vi "ClassPanel.vi"(8 "error in (no error)":errorcluster caption="entrée d'erreur (pas d'erreur)", 11 "SR830.lvclass":refnum<class "SR830.lvclass">) -> (0 "error out":errorcluster caption="sortie d'erreur", 3 "SR830.lvclass Out":refnum<class "SR830.lvclass">)   [LabVIEW 2019, in "SR830.lvclass"]
uses:
  SR830.lvclass
  C:/Programmes Labview/LabScanV1A/DevicesClass/BaseDevice/BaseDevice.lvclass
  BaseDevice/BaseDevice.lvclass/BaseDevice.ctl
  BaseDevice/Accessor/GetBeforewait(ms).vi
  BaseDevice/Accessor/GetClassEvent.vi
  BaseDevice/Accessor/SetBeforewait.vi
panel:
  in  "MainProgQ":refnum<queue>
  in  "MainProgQEvent":refnum<user-event>
  in  "Time Constant":u16(ring)=1 items=["10 us", "30 us", "100 us", "300 us", "1 ms", "3 ms", "10 ms", "30 ms", "100 ms", "300 ms", "1 s", "3 s", "10 s", "30 s", "100 s", "300 s", "1 ks", "3 ks", "10 ks", "30 ks"]
  in  "BefWait (ms)":u32 caption="BeforeWait Delay(ms)" max=200000 step=1
  in  "Sensitivity":u16(ring)=1 items=["2 nV/fA", "5 nV/fA", "10 nV/fA", "20 nV/fA", "50 nV/fA", "100 nV/fA", "200 nV/fA", "500 nV/fA", "1 µV/pA", "2 µV/pA", "5 µV/pA", "10 µV/pA", "20 µV/pA", "50 µV/pA", "100µV/pA", "200 µV/pA", "500µV/pA", "1 mV/nA", "2 mV/nA", "5 mV/nA", "10 mV/nA", "20 mV/nA", "50 mV/nA", "100 mV/nA", "200 mV/nA", "500 mV/nA", "1 V/uA"]
  in  "Acq":bool
  out "Phase":dbl=1000.0 caption="Phase (°)" min=0.0 step=0.1 format="%#_5f"
  out "MAG":dbl=1000.0 caption="MAG (V)" min=0.0 step=0.1 format="%^#_6e"
  out "UNLCK":bool caption="SpexMov"
  out "X":dbl=1000.0 caption="X (V)" min=0.0 step=0.1 format="%^#_6e"
  in  "Stop":bool
  out "Init Program":bool
  out "OVLD":bool caption="SpexMov"
  in  "Update":bool caption="stopSpectro"
  out "Y":dbl=1000.0 caption="Y (V)" min=0.0 step=0.1 format="%^#_6e"
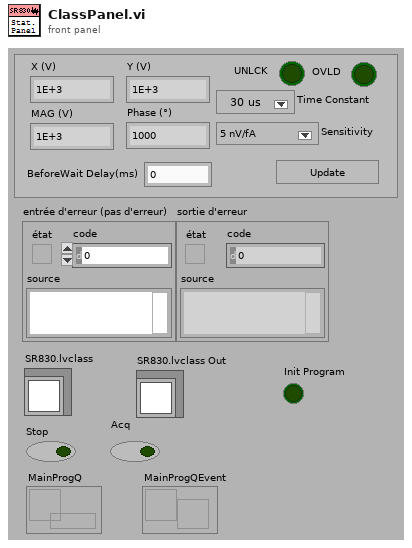
[diagram p1: front panel]
types:
  T1 = enum16{"Phase Shift", "Reference Source", "Reference Frequency", "Reference Trigger", "Detection Harmonic", "Sine Amplitude", "Input Configuration", "Input Shield", "Input Coupling", "Input Line Notch Filter", "Sensitivity", "Dynamic Reserve", "Time Constant", "Low Pass Filter", "Sync Filter", "Expand X", "Expand Y", "Expand R", "All"}
  T2 = enum16{"Sensitivity", "Dynamic Reserve", "Time Constant"}
  T3 = cluster{"Channels":u16, "Outputs":dbl[], "Status Byte":bool[]}
  T4 = enum8{"Enabled", "Disabled", "Disabled and Grayed Out"}
  T5 = cluster{"Phase Shift (°)":dbl, "Reference Source":u16, "Frequency (Hz)":dbl, "Reference Trigger":u16, "Harmonic":i32, "Sine Amplitude (V)":dbl, "Input Configuration":u16, "Input Shield":u16, "Input Coupling":u16, "Input Notch Filters":cluster{"1xLineFilter":bool, "2xLineFilter":bool}, "Sensitivity":u16, "Dynamic Reserve":u16, "Time Constant":u16, "Low Pass Filter":u16, "Sync Filter":bool, "Expand X":cluster{"Offset (%)":dbl, "Expand":u16}, "Expand Y":cluster{"Offset (%)":dbl, "Expand":u16}, "Expand R":cluster{"Offset (%)":dbl, "Expand":u16}}
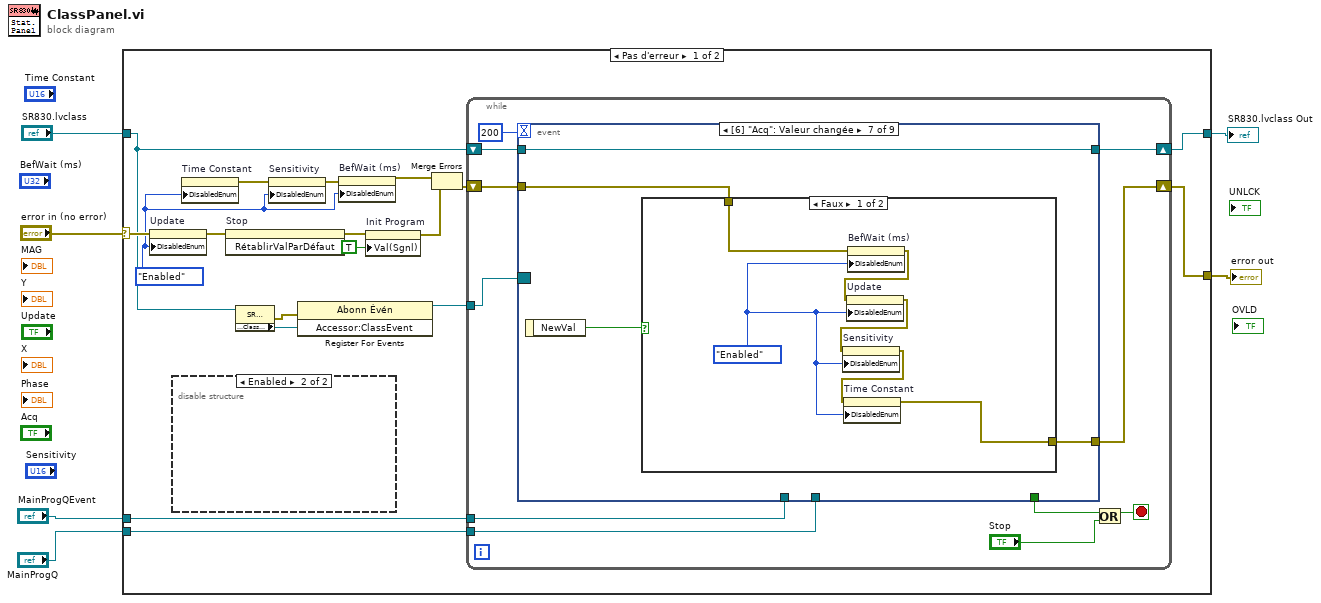
[diagram p0: block diagram]
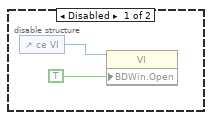
[diagram p2: hidden frame]
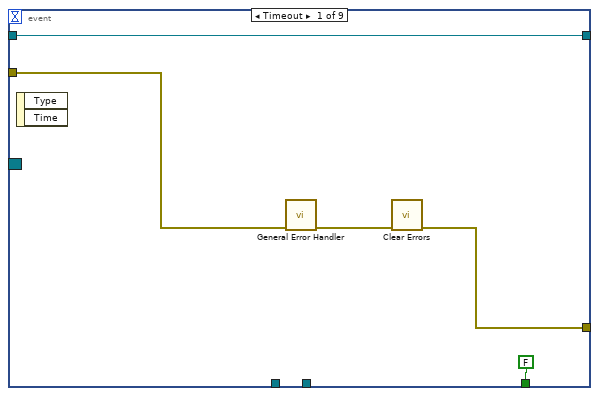
[diagram p3: hidden frame]
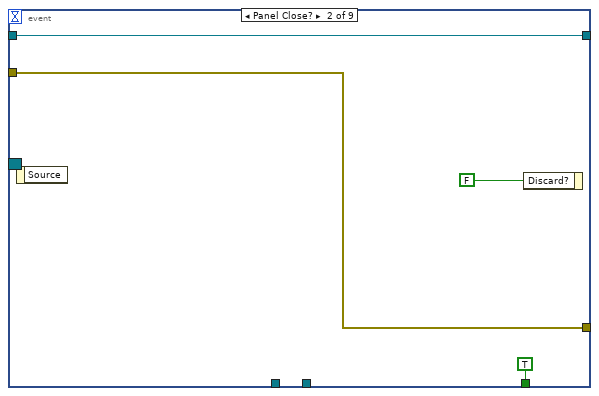
[diagram p4: hidden frame]
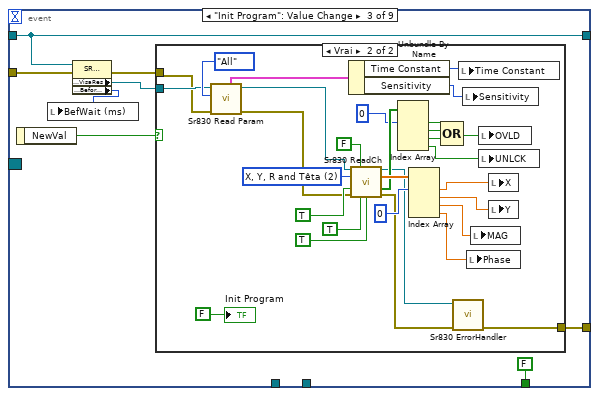
[diagram p5: hidden frame]
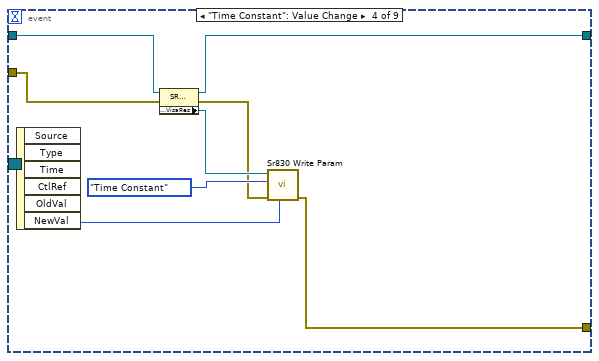
[diagram p7: hidden frame]
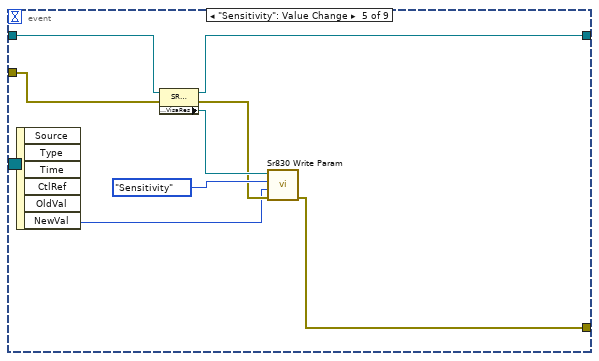
[diagram p8: hidden frame]
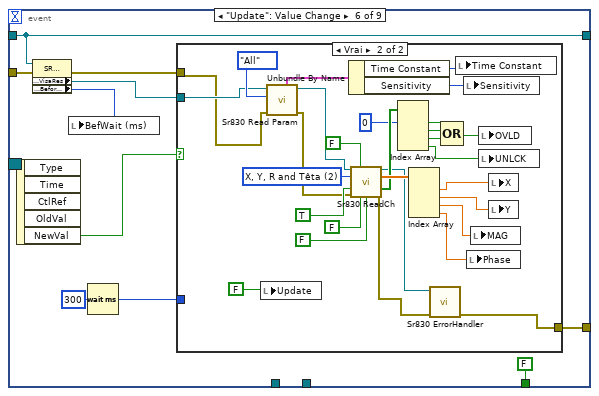
[diagram p9: hidden frame]
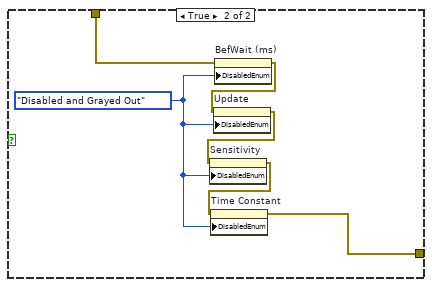
[diagram p11: hidden frame]
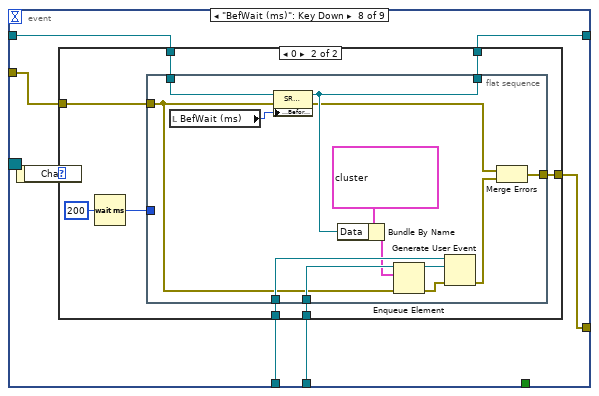
[diagram p12: hidden frame]
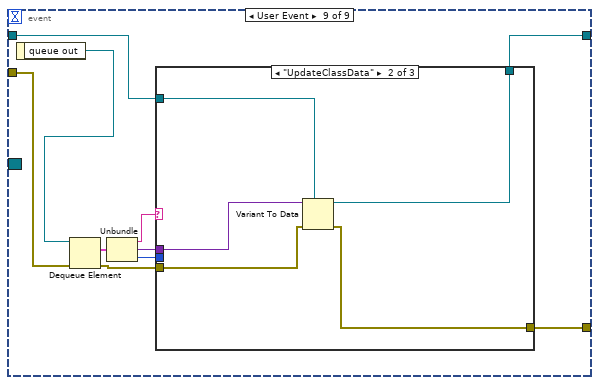
[diagram p14: hidden frame]
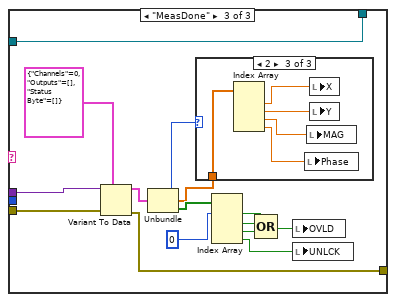
[diagram p16: hidden frame]
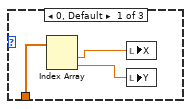
[diagram p17: hidden frame]
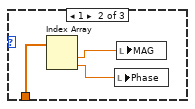
[diagram p18: hidden frame]
diagram:
  n1 = case shown="Pas d'erreur" "error in (no error)" {
    selector: "error in (no error)" -> [w21 w231]
    tunnel: [w16 w231] -> w5
    tunnel: "SR830.lvclass" -> [w14 w230]
    tunnel: [w23 w230] -> w3
    tunnel: "MainProgQEvent" -> [w13 _]
    tunnel: "MainProgQ" -> [w12 _]
    frame No Error {
      w7 = T4."Enabled" ("Désactivé")
      n2 = property on="Update" class="Bool (strict)"(error in=w21, "DisabledEnum"=w7) -> (error out=w18:errorcluster)  [unwired: 1 in, 1 out]
      n3 = disable-structure shown="Enabled" {
        frame Disabled {
          n4 = control-ref of="ce VI"() -> (w26:refnum<vi>)
          n5 = property class="VI"(reference=w26, "BDWin.Open"=TRUE ("Fenêtre du diagramme : ouverte")) -> ()  [unwired: 1 in, 2 out]
        }
        frame Enabled {
        }
      }
      n6 = property on="Time Constant" class="MDér (strict)"("DisabledEnum"=w7) -> (error out=w11:errorcluster)  [unwired: 2 in, 1 out]
      n7 = invoke on="Stop" class="Bool (strict)" method="RétablirValParDéfaut"(error in=w18) -> (error out=w22:errorcluster)  [unwired: 2 in, 2 out]
      n8 = property class="SR830.lvclass"(reference=w14) -> (error out=w19:errorcluster, "Accessor:ClassEvent"=w20:refnum<user-event>)  [unwired: 1 in, 1 out]
      n9 = property on="Sensitivity" class="MDér (strict)"(error in=w11, "DisabledEnum"=w7) -> (error out=w10:errorcluster)  [unwired: 1 in, 1 out]
      n10 = register-events(error in=w19, w20) -> (reference out=w17:refnum<event-registration>)  [unwired: 1 in, 1 out]
      n11 = property on="BefWait (ms)" class="NumNb (strict)"(error in=w10, "DisabledEnum"=w7) -> (error out=w8:errorcluster)  [unwired: 1 in, 1 out]
      n12 = property on="Init Program" class="Bool (strict)"(error in=w22, "Val(Sgnl)"=TRUE ("Valeur (Signalisation)")) -> (error out=w15:errorcluster)  [unwired: 1 in, 1 out]
      n13 = Merge Errors(w8, w15) -> (w9:errorcluster)
      n14 = while {
        shift-right: [w35] -> w16
        shift-left: w9 -> [w36]
        shift-right: [w32] -> w23
        shift-left: w14 -> [w34]
        tunnel: w17 -> [w29]
        tunnel: w13 -> [w28]
        tunnel: w12 -> [w27]
        stop <- w31 stop-if-true
        n15 = event shown="[6] \"Acq\": Valeur changée" {
          selector: w29 -> [_ _ _ _ _ _ _ _ _]
          dyn-events: _ -> [_ _ _ _ _ _ _ _ _]
          timeout: 200 -> [_ _ _ _ _ _ _ _ _]
          tunnel: w36 -> [w40 w44 w52 w91 w99 w105 w144 w161 w194]
          tunnel: [w38 w44 w51 w87 w95 w109 w142 w160 w188] -> w35
          tunnel: w34 -> [w41 w43 w49 w92 w100 w104 w141 w163 w191]
          tunnel: [FALSE TRUE FALSE _ _ FALSE _ _ _] -> w33
          tunnel: [w41 w43 w49 w86 w94 w104 w141 w162 w190] -> w32
          tunnel: w28 -> [_ _ _ _ _ _ _ w159 _]
          tunnel: w27 -> [_ _ _ _ _ _ _ w158 _]
          event Timeout {
            n16 = event-data() -> ()  [unwired: 1 in, 2 out]
            n17 = call <vilib>:"General Error Handler.vi"("error in (no error)"=w40) -> ("error out"=w39:errorcluster)  [unwired: 10 in, 4 out]
            n18 = call <vilib>:"Clear Errors.vi"("error in (no error)"=w39) -> ("error out"=w38:errorcluster)  [unwired: 5 in, 1 out]
          }
          event Panel Close? {
            n19 = event-data() -> ()  [unwired: 1 in, 1 out]
            n20 = event-data("Discard?"=FALSE ("Rejeter ?")) -> ()  [unwired: 1 in, 1 out]
          }
          event "Init Program": Value Change {
            n21 = event-data() -> ("NewVal"=w53:bool)  [unwired: 1 in]
            n22 = property class="SR830.lvclass"(reference=w49) -> ("Accessor:VisaRes"=w48:refnum<visa-resource-name>, "Accessor:Beforewait(ms)"=w47:u32)  [unwired: 1 in, 2 out]
            n23 = local write "BefWait (ms)"(w47) -> ()
            n24 = case shown="Vrai" w53 {
              tunnel: w48 -> [_ w68]
              tunnel: w52 -> [w54 w61]
              tunnel: [w54 w59] -> w51
              frame False {
              }
              frame True {
                w76 = u16 2 items=["X and Y", "R and Têta", "X, Y, R and Têta"] ("Channels")
                n25 = call <userlib>:"Sr830 Read Param.vi"("error in (no error)"=w61, "Énum"=T1."All", "Ressource VISA"=w68) -> ("error out"=w60:errorcluster, "Ressource VISA Out"=w67:refnum<visa-resource-name>, "LockInPar"=w66:T5)  [unwired: 5 in, 1 out]
                n26 = Unbundle By Name(w66) -> ("Time Constant"=w55:u16, "Sensitivity"=w56:u16)
                n27 = call <userlib>:"Sr830 ReadCh.vi"("VISA Rsrc"=w67, "Autoscale"=FALSE, "Channels"=w76, "Check Status"=TRUE, "error in (no error)"=w60, "Ask Correction"=TRUE, "Show Warning"=TRUE) -> ("Ressource VISA Out"=w58:refnum<visa-resource-name>, "Outputs"=w83:dbl[], "Status Byte"=w82:bool[], "error out"=w57:errorcluster)  [unwired: 3 in, 2 out]
                n28 = Index Array(array=w82, index #1=0 ("indice")) -> (element #1=w73:bool, element #2=w72:bool, element #3=w71:bool, element #4=w74:bool)  [unwired: 3 in]
                n29 = Index Array(array=w83, index #1=0 ("indice")) -> (element #1=w81:dbl, element #2=w80:dbl, element #3=w79:dbl, element #4=w78:dbl)  [unwired: 3 in]
                n30 = Compound Arithmetic op=OR(w73, w72, w71) -> (w70:bool)
                n31 = call <userlib>:"Sr830 ErrorHandler.vi"("error in (no error)"=w57, "VisaRes"=w58) -> ("error out"=w59:errorcluster)  [unwired: 8 in, 1 out]
                n32 = local write "Time Constant"(w55) -> ()
                n33 = local write "Sensitivity"(w56) -> ()
                n34 = local write "Phase"(w78) -> ()
                n35 = local write "MAG"(w79) -> ()
                n36 = local write "OVLD"(w70) -> ()
                n37 = local write "UNLCK"(w74) -> ()
                n38 = local write "X"(w81) -> ()
                n39 = local write "Y"(w80) -> ()
                "Init Program" <- FALSE
              }
            }
          }
          event "Time Constant": Value Change {
            n40 = event-data() -> ("NewVal"=w85:u16)  [unwired: 1 in, 5 out]
            n41 = property class="SR830.lvclass"(reference=w92, error in=w91) -> (reference out=w86:refnum<class "SR830.lvclass">, error out=w88:errorcluster, "Accessor:VisaRes"=w90:refnum<visa-resource-name>)
            n42 = call <userlib>:"Sr830 Write Param.vi"("Time Constant"=w85, "error in"=w88, "Param"=T2."Time Constant", "Ressource VISA"=w90) -> ("error out"=w87:errorcluster)  [unwired: 6 in, 1 out]
          }
          event "Sensitivity": Value Change {
            n43 = event-data() -> ("NewVal"=w93:u16)  [unwired: 1 in, 5 out]
            n44 = property class="SR830.lvclass"(reference=w100, error in=w99) -> (reference out=w94:refnum<class "SR830.lvclass">, error out=w96:errorcluster, "Accessor:VisaRes"=w98:refnum<visa-resource-name>)
            n45 = call <userlib>:"Sr830 Write Param.vi"("error in"=w96, "Sensitivity"=w93, "Param"=T2."Sensitivity", "Ressource VISA"=w98) -> ("error out"=w95:errorcluster)  [unwired: 6 in, 1 out]
          }
          event "Update": Value Change {
            n46 = event-data() -> ("NewVal"=w110:bool)  [unwired: 1 in, 4 out]
            n47 = property class="SR830.lvclass"(reference=w104, error in=w105) -> (error out=w103:errorcluster, "Accessor:VisaRes"=w102:refnum<visa-resource-name>, "Accessor:Beforewait(ms)"=w101:u32)  [unwired: 1 out]
            n48 = local write "BefWait (ms)"(w101) -> ()
            n49 = Wait (ms)(milliseconds to wait=u32 300 ("attente (ms)")) -> (millisecond timer value=w106:u32)
            n50 = case shown="Vrai" w110 {
              tunnel: w102 -> [_ w125]
              tunnel: w103 -> [w111 w119]
              tunnel: [w111 w115] -> w109
              tunnel: w106 -> [_ _]
              frame False {
              }
              frame True {
                w133 = u16 2 items=["X and Y", "R and Têta", "X, Y, R and Têta"] ("Channels")
                n51 = local write "Update"(FALSE) -> ()
                n52 = call <userlib>:"Sr830 Read Param.vi"("error in (no error)"=w119, "Énum"=T1."All", "Ressource VISA"=w125) -> ("error out"=w118:errorcluster, "Ressource VISA Out"=w124:refnum<visa-resource-name>, "LockInPar"=w123:T5)  [unwired: 5 in, 1 out]
                n53 = Unbundle By Name(w123) -> ("Time Constant"=w112:u16, "Sensitivity"=w122:u16)
                n54 = call <userlib>:"Sr830 ReadCh.vi"("VISA Rsrc"=w124, "Autoscale"=FALSE, "Channels"=w133, "Check Status"=TRUE, "error in (no error)"=w118, "Ask Correction"=FALSE, "Show Warning"=FALSE) -> ("Ressource VISA Out"=w114:refnum<visa-resource-name>, "Outputs"=w140:dbl[], "Status Byte"=w139:bool[], "error out"=w113:errorcluster)  [unwired: 3 in, 2 out]
                n55 = Index Array(array=w139, index #1=0 ("indice")) -> (element #1=w130:bool, element #2=w129:bool, element #3=w128:bool, element #4=w131:bool)  [unwired: 3 in]
                n56 = Index Array(array=w140) -> (element #1=w138:dbl, element #2=w137:dbl, element #3=w136:dbl, element #4=w135:dbl)  [unwired: 4 in]
                n57 = call <userlib>:"Sr830 ErrorHandler.vi"("error in (no error)"=w113, "VisaRes"=w114) -> ("error out"=w115:errorcluster)  [unwired: 8 in, 1 out]
                n58 = Compound Arithmetic op=OR(w130, w129, w128) -> (w127:bool)
                n59 = local write "Time Constant"(w112) -> ()
                n60 = local write "Sensitivity"(w122) -> ()
                n61 = local write "Phase"(w135) -> ()
                n62 = local write "MAG"(w136) -> ()
                n63 = local write "OVLD"(w127) -> ()
                n64 = local write "UNLCK"(w131) -> ()
                n65 = local write "X"(w138) -> ()
                n66 = local write "Y"(w137) -> ()
              }
            }
          }
          event "Acq": Value Change {
            n67 = event-data() -> ("NewVal"=w143:bool)  [unwired: 1 in]
            n68 = case shown="Faux" w143 {
              tunnel: w144 -> [w149 w155]
              tunnel: [w146 w152] -> w142
              frame False {
                w145 = T4."Enabled" ("Désactivé")
                n69 = property on="BefWait (ms)" class="NumNb (strict)"(error in=w149, "DisabledEnum"=w145) -> (error out=w150:errorcluster)  [unwired: 1 in, 1 out]
                n70 = property on="Update" class="Bool (strict)"(error in=w150, "DisabledEnum"=w145) -> (error out=w148:errorcluster)  [unwired: 1 in, 1 out]
                n71 = property on="Sensitivity" class="MDér (strict)"(error in=w148, "DisabledEnum"=w145) -> (error out=w147:errorcluster)  [unwired: 1 in, 1 out]
                n72 = property on="Time Constant" class="MDér (strict)"(error in=w147, "DisabledEnum"=w145) -> (error out=w146:errorcluster)  [unwired: 1 in, 1 out]
              }
              frame True {
                w151 = T4."Disabled and Grayed Out" ("Désactivé")
                n73 = property on="BefWait (ms)" class="NumNb (strict)"(error in=w155, "DisabledEnum"=w151) -> (error out=w156:errorcluster)  [unwired: 1 in, 1 out]
                n74 = property on="Update" class="Bool (strict)"(error in=w156, "DisabledEnum"=w151) -> (error out=w154:errorcluster)  [unwired: 1 in, 1 out]
                n75 = property on="Sensitivity" class="MDér (strict)"(error in=w154, "DisabledEnum"=w151) -> (error out=w153:errorcluster)  [unwired: 1 in, 1 out]
                n76 = property on="Time Constant" class="MDér (strict)"(error in=w153, "DisabledEnum"=w151) -> (error out=w152:errorcluster)  [unwired: 1 in, 1 out]
              }
            }
          }
          event "BefWait (ms)": Key Down {
            n77 = event-data() -> ("Char"=w157:i16)  [unwired: 1 in]
            n78 = case shown="0" w157 {
              tunnel: w163 -> [w165 w173]
              tunnel: [w165 w172] -> w162
              tunnel: w161 -> [w164 w169]
              tunnel: [w164 w168] -> w160
              tunnel: w159 -> [_ w171]
              tunnel: w158 -> [_ w170]
              frame Default {
              }
              frame 0 {
                n79 = Wait (ms)(milliseconds to wait=u32 200 ("attente (ms)")) -> (millisecond timer value=w166:u32)
                n80 = flat-sequence {
                  tunnel: w173 -> [w185]
                  tunnel: [w183] -> w172
                  tunnel: w171 -> [w179]
                  tunnel: w170 -> [w178]
                  tunnel: w169 -> [w177]
                  tunnel: [w176] -> w168
                  tunnel: w166 -> [_]
                  frame #0 {
                    n81 = local read "BefWait (ms)"() -> (w184:u32)
                    n82 = property class="SR830.lvclass"(reference=w185, error in=w177, "Accessor:Beforewait(ms)"=w184) -> (reference out=w183:refnum<class "SR830.lvclass">, error out=w182:errorcluster)
                    n83 = Bundle By Name(cluster=cluster{"Message":string, "Data":variant, i32} {"Message"="UpdateMainClass", "Data"=variant, 0} ("élément"), "Data"=w183) -> (w174:cluster{"Message":string, "Data":variant, i32})
                    n84 = Enqueue Element(queue=w178, element=w174, error in (no error)=w177) -> (queue out=w180:refnum<queue>, error out=w181:errorcluster)  [unwired: 1 in, 1 out]
                    n85 = Generate User Event(user event=w179, event data cluster=w180, error in=w181) -> (error out=w175:errorcluster)  [unwired: 1 in, 1 out]
                    n86 = Merge Errors(w182, w175) -> (w176:errorcluster)
                  }
                }
              }
            }
          }
          event User Event {
            n87 = event-data() -> ("queue out"=w195:refnum<queue>)  [unwired: 1 in]
            n88 = Dequeue Element(queue=w195, error in (no error)=w194) -> (element=w196:cluster{"Message":string, "Data":variant, i32}, error out=w189:errorcluster)  [unwired: 1 in, 2 out]
            n89 = Unbundle(w196) -> ("Message"=w187:string, "Data"=w193:variant, w192:i32)
            n90 = case shown="\"UpdateClassData\"" w187 {
              tunnel: w193 -> [_ w201 w218]
              tunnel: w192 -> [_ _ _]
              tunnel: w191 -> [w198 w203 w208]
              tunnel: [w198 w202 w208] -> w190
              tunnel: w189 -> [w197 w200 w217]
              tunnel: [w197 w199 w216] -> w188
              frame Default {
              }
              frame "UpdateClassData" {
                n91 = Variant To Data(error in=w200, type=w203, Variant=w201) -> (data=w202:refnum<class "SR830.lvclass">, error out=w199:errorcluster)
              }
              frame "MeasDone" {
                n92 = Variant To Data(error in=w217, type=T3 {"Channels"=0, "Outputs"=[], "Status Byte"=[]} ("cluster"), Variant=w218) -> (data=w215:T3, error out=w216:errorcluster)
                n93 = Unbundle(w215) -> ("Channels"=w204:u16, "Outputs"=w205:dbl[], "Status Byte"=w206:bool[])
                n94 = case shown="2" w204 {
                  tunnel: w205 -> [w219 w222 w229]
                  frame 0, Default {
                    n95 = Index Array(array=w219) -> (element #1=w221:dbl, element #2=w220:dbl)  [unwired: 2 in]
                    n96 = local write "X"(w221) -> ()
                    n97 = local write "Y"(w220) -> ()
                  }
                  frame 1 {
                    n98 = Index Array(array=w222) -> (element #1=w224:dbl, element #2=w223:dbl)  [unwired: 2 in]
                    n99 = local write "Phase"(w223) -> ()
                    n100 = local write "MAG"(w224) -> ()
                  }
                  frame 2 {
                    n101 = Index Array(array=w229) -> (element #1=w226:dbl, element #2=w225:dbl, element #3=w228:dbl, element #4=w227:dbl)  [unwired: 4 in]
                    n102 = local write "Phase"(w227) -> ()
                    n103 = local write "MAG"(w228) -> ()
                    n104 = local write "X"(w226) -> ()
                    n105 = local write "Y"(w225) -> ()
                  }
                }
                n106 = Index Array(array=w206, index #1=0 ("indice")) -> (element #1=w213:bool, element #2=w212:bool, element #3=w211:bool, element #4=w214:bool)  [unwired: 3 in]
                n107 = Compound Arithmetic op=OR(w213, w212, w211) -> (w210:bool)
                n108 = local write "OVLD"(w210) -> ()
                n109 = local write "UNLCK"(w214) -> ()
              }
            }
          }
        }
        n110 = Or(x=w33, y="Stop") -> (x .or. y?=w31:bool)
      }
    }
    frame Error {
    }
  }
  "error out" <- w5
  "SR830.lvclass Out" <- w3
